vi "Previous Page.vi"(8 "error in (no error)":errorcluster, 11 "Project Model in":refnum<class "Project Model.lvclass">) -> (0 "error out":errorcluster, 3 "Project Model out":refnum<class "Project Model.lvclass">)   [LabVIEW 2013, in "Project Model.lvlib" / "Project Model.lvclass"]
uses:
  Project Model.lvclass
  Project Model.lvclass/Project Model.ctl
  <vilib>/ActorFrameworkMVC/View Observer/View Registry/View Registry.lvclass/View Registry.ctl
  Project Model Messages/Abstract Move In Previous Msg/Abstract Move In Previous Msg.lvclass
  <vilib>/ActorFrameworkMVC/View Observer/Data Message/Data Message.lvclass
  <vilib>/ActorFrameworkMVC/View Observer/View Registry/View Registry.lvclass
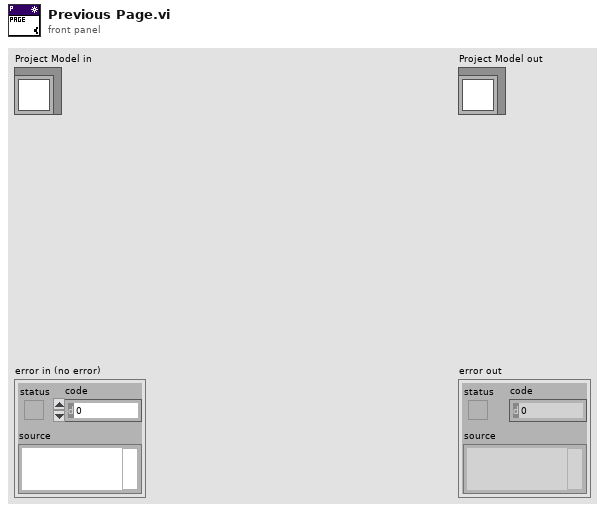
[diagram p1: front panel]
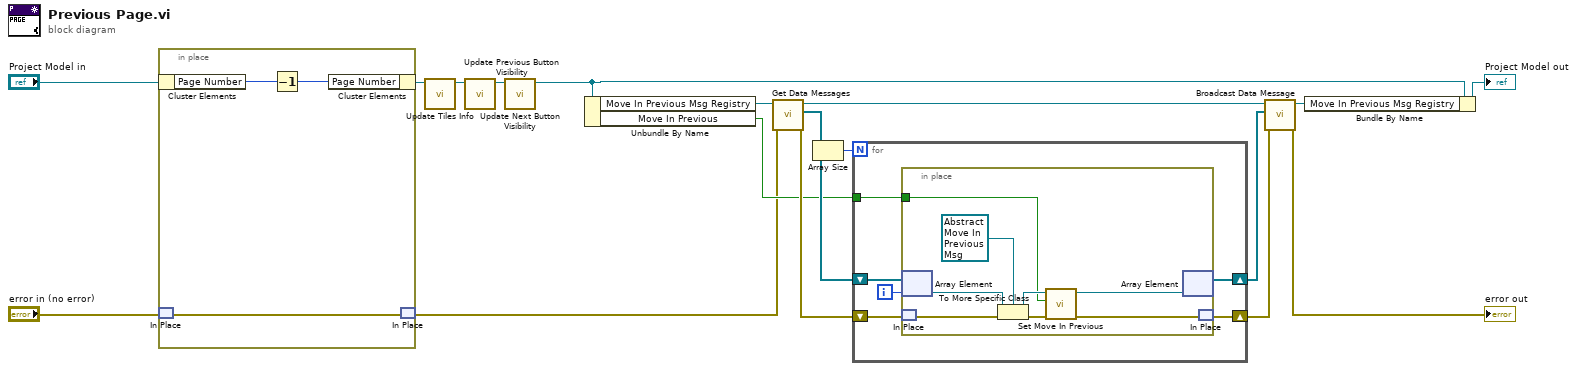
[diagram p0: block diagram]
diagram:
  n1 = in-place {
    n2 = in-place-cluster #1("Project Model in") -> ("Page Number"=w21:i32)
    n3 = in-place-match #2("error in (no error)") -> (w19:errorcluster)
    n4 = Decrement(x=w21) -> (x-1=w20:i32)
    n5 = in-place-cluster #1("Page Number"=w20) -> (w7:refnum<class "Project Model.lvclass">)
    n6 = in-place-match #2(w19) -> (w4:errorcluster)
  }
  n7 = call "Update Tiles Info.vi"("Project Model in"=w7) -> ("Project Model out"=w3:refnum<class "Project Model.lvclass">)  [unwired: 9 in, 1 out]
  n8 = call "Update Previous Button Visibility.vi"("Project Model in"=w3) -> ("Project Model out"=w2:refnum<class "Project Model.lvclass">)  [unwired: 9 in, 1 out]
  n9 = call "Update Next Button Visibility.vi"("Project Model in"=w2) -> ("Project Model out"=w1:refnum<class "Project Model.lvclass">)  [unwired: 9 in, 1 out]
  n10 = Unbundle By Name(w1) -> ("Move In Previous Msg Registry"=w16:refnum<class "View Registry.lvclass">, "Move In Previous"=w8:bool)
  n11 = call <vilib>:"Get Data Messages.vi"("error in (no error)"=w4, "View Registry in"=w16) -> ("error out"=w12:errorcluster, "Data Messages"=w13:refnum<class "Data Message.lvclass">[], "View Registry out"=w15:refnum<class "View Registry.lvclass">)  [unwired: 7 in]
  n12 = Array Size(array=w13) -> (size(s)=w14:i32)
  n13 = for {
    N: w14 -> [_]
    shift-right: [w26] -> w11
    shift-left: w13 -> [w27]
    shift-right: [w23] -> w10
    shift-left: w12 -> [w25]
    tunnel: w8 -> [w24]
    i -> [w22]
    n14 = in-place {
      in-place-border: w24 -> [w28]
      n15 = in-place-array #3(w27, w22) -> (w33:refnum<class "Data Message.lvclass">)
      n16 = in-place-match #4(w25) -> (w35:errorcluster)
      n17 = To More Specific Class(target class=refnum<class "Abstract Move In Previous Msg.lvclass"> refnum ("Project Model.lvlib:Abstract Move In Previous Msg.lvclass"), reference=w33, error in=w35) -> (specific class reference=w29:refnum<class "Abstract Move In Previous Msg.lvclass">, error out=w32:errorcluster)
      n18 = call "Set Move In Previous.vi"("error in (no error)"=w32, "Move In Previous"=w28, "Abstract Move In Previous Msg in"=w29) -> ("error out"=w31:errorcluster, "Abstract Move In Previous Msg out"=w30:refnum<class "Abstract Move In Previous Msg.lvclass">)  [unwired: 7 in]
      n19 = in-place-array #3(w30) -> (w26:refnum<class "Data Message.lvclass">[])  [unwired: 1 out]
      n20 = in-place-match #4(w31) -> (w23:errorcluster)
    }
  }
  n21 = call <vilib>:"Broadcast Data Message.vi"("error in (no error)"=w10, "Data Messages"=w11, "View Registry in"=w15) -> ("error out"=→"error out":errorcluster, "View Registry out"=w9:refnum<class "View Registry.lvclass">)  [unwired: 7 in]
  n22 = Bundle By Name(cluster=w1, "Move In Previous Msg Registry"=w9) -> (→"Project Model out":refnum<class "Project Model.lvclass">)
